vi "poly_linspace_FXP.vi"(6 "inclusive? (T)":bool=TRUE, 8 "xN":fxp<+/-,64,32>, 9 "N":i32, 10 "x0":fxp<+/-,64,32>) -> (1 "linspace out":fxp<+/-,64,32>[](array[numeric]))   [LabVIEW 2015]
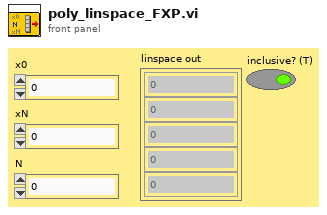
[diagram p1: front panel]
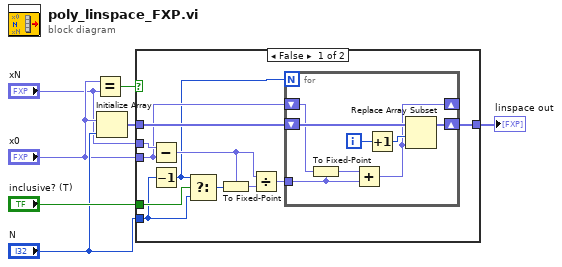
[diagram p0: block diagram]
diagram:
  n1 = Equal?(x="x0", y="xN") -> (x = y?=w1:bool)
  n2 = Initialize Array("x0", "N") -> (w7:fxp<+/-,64,32>[])
  n3 = case shown="False" w1 {
    tunnel: w7 -> [w18 w27]
    tunnel: [w17 w27] -> w6
    tunnel: "xN" -> [w16 _]
    tunnel: "x0" -> [w14 _]
    tunnel: "inclusive? (T)" -> [w13 _]
    tunnel: "N" -> [w8 _]
    frame False {
      n4 = Subtract(x=w16, y=w14) -> (x-y=w11:fxp<+/-,64,33>)
      n5 = Decrement(x=w8) -> (x-1=w9:i32)
      n6 = Select(t=w9, s=w13, f=w8) -> (s? t:f=w10:i32)
      n7 = To Fixed-Point(fixed-point type=w11, number=w10) -> (fixed-point=w12:fxp<+/-,64,33>)
      n8 = Divide(x=w11, y=w12) -> (x/y=w15:fxp<+/-,64,65>)
      n9 = for {
        N: w9 -> [_]
        shift-right: [w25] -> w17
        shift-left: w18 -> [w26]
        shift-right: [w22] -> _
        shift-left: w14 -> [w20]
        tunnel: w15 -> [w21]
        i -> [w24]
        n10 = To Fixed-Point(fixed-point type=w21, number=w20) -> (fixed-point=w19:fxp<+/-,64,65>)
        n11 = Add(x=w19, y=w21) -> (x+y=w22:fxp<+/-,64,66>)
        n12 = Increment(x=w24) -> (x+1=w23:i32)
        n13 = Replace Array Subset(array=w26, new element=w22, index=w23) -> (w25:fxp<+/-,64,32>[])
      }
    }
    frame True {
    }
  }
  "linspace out" <- w6
